vi "set RT Stop.vi"(8 "error in (no error)":errorcluster, 11 "RT Stop":bool) -> (0 "error out":errorcluster)   [LabVIEW 2024]
uses:
  cRIO VI parameters.vi
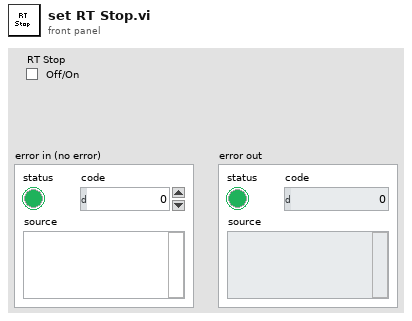
[diagram p1: front panel]
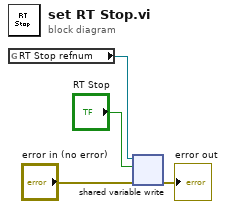
[diagram p0: block diagram]
diagram:
  n1 = global read "cRIO VI parameters.vi" "RT Stop refnum"() -> (w1:refnum<k21>)
  n2 = shared-variable-write(w1, "error in (no error)", "RT Stop") -> (→"error out":errorcluster)  [unwired: 1 out]
